vi "armsim-arm-ctrl-init.vi"(11 "Linearsystem":T4) -> (0 "Kalman Error":errorcluster, 1 "KalmanFilter":T3, 2 "LinSysLoopError":bool, 3 "Linear System Loop":T5, 4 "LinearQuadraticRegulator":T1, 6 "Lqr Error":bool)   [LabVIEW 2019]
uses:
  <vilib>/Rock Robotics/WPI/ThirdParty/JAS_Junk/TrajLib/TypeDef/LINEAR_SYSTEM.ctl
  <vilib>/Analysis/Matrix/Datatypes/RealMatrix.ctl
  <vilib>/Rock Robotics/WPI/ThirdParty/JAS_Junk/TrajLib/TypeDef/LINEAR_SYSTEM_LOOP.ctl
  <vilib>/Rock Robotics/WPI/ThirdParty/JAS_Junk/TrajLib/TypeDef/LINEAR_QUADRATIC_REGULATOR.ctl
  <vilib>/Rock Robotics/WPI/ThirdParty/JAS_Junk/TrajLib/TypeDef/LINEAR_PLANT_INV_FF.ctl
  <vilib>/Rock Robotics/WPI/ThirdParty/JAS_Junk/TrajLib/TypeDef/KALMAN_FILTER.ctl
  <vilib>/Rock Robotics/WPI/ThirdParty/JAS_Junk/TrajLib/MatBuilder_Create.vi
  <vilib>/Rock Robotics/WPI/ThirdParty/JAS_Junk/TrajLib/Trajectory_Library.lvlib
  <vilib>/Analysis/Matrix/NI_Matrix.lvlib
panel:
  # "Ref State <States,1>"
  # "Comp and capped \noutput <Inputs,1>"
  # "Controller gain\n<Inputs,States>"
  # "Steady State Gain  \n<States,Outputs>"
  # "State Estimate <Statess,1>"
  # "<States,States>"
  # "<States,Inputs>"
  # "<Outputs,States>"
  # "<Outputs,Inputs>"
  # "<States,1>"
  # "<FUTURE --- CLAMP TYPE -- For now\nuse Normalize>"
  # "Steady State Gain  \n<States,Outputs>"
  # "State Estimate <Statess,1>"
  # "<States,States>"
  # "<States,Inputs>"
  # "<Outputs,States>"
  # "<Outputs,Inputs>"
  # "<States,1>"
  # "<Inputs,1>"
  # "<States,Inputs>"
  # "<States,States>"
  # "Ref State <States,1>"
  # "Comp and capped \noutput <Inputs,1>"
  # "Controller gain\n<Inputs,States>"
  # "<States,States>"
  # "<States,Inputs>"
  # "<Outputs,States>"
  # "<Outputs,Inputs>"
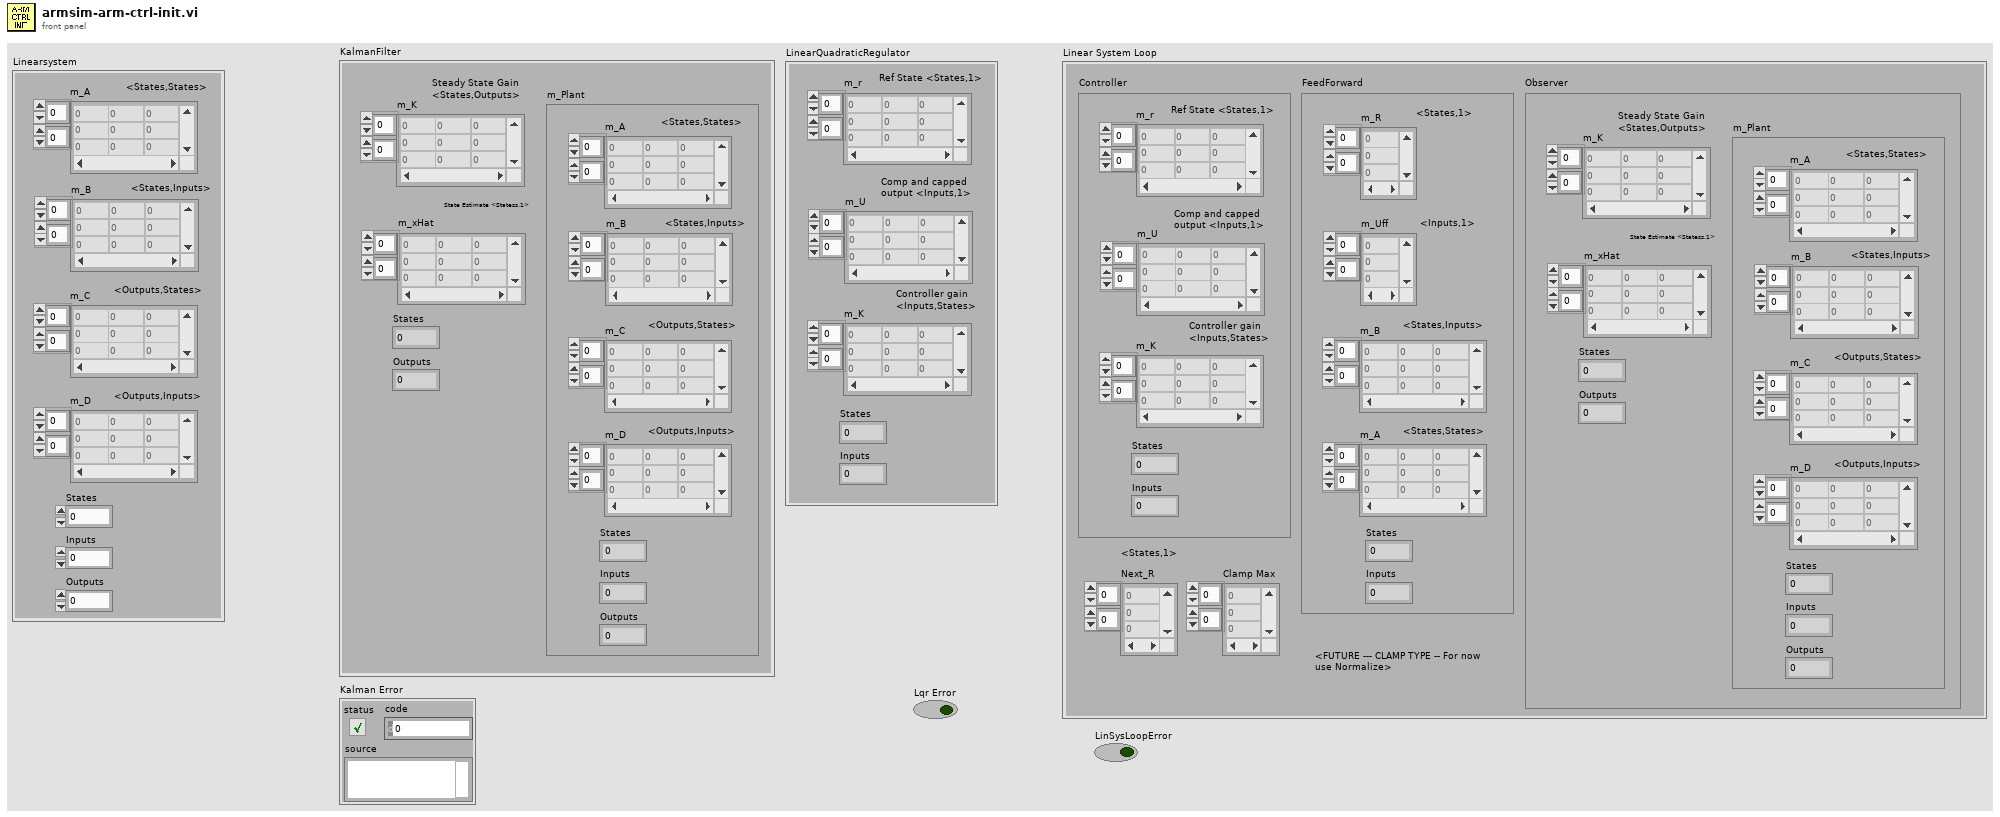
[diagram p1: front panel]
types:
  T1 = typedef "Trajectory_Library.lvlib/LINEAR_QUADRATIC_REGULATOR.ctl" = cluster{"m_r":T2, "m_U":T2, "m_K":T2, "States":i32, "Inputs":i32}
  T2 = typedef "NI_Matrix.lvlib/RealMatrix.ctl" = dbl[][]
  T3 = typedef "Trajectory_Library.lvlib/KALMAN_FILTER.ctl" = cluster{"m_K":T2, "m_xHat":T2, "States":i32, "Outputs":i32, "m_Plant":T4}
  T4 = typedef "Trajectory_Library.lvlib/LINEAR_SYSTEM.ctl" = cluster{"m_A":T2, "m_B":T2, "m_C":T2, "m_D":T2, "States":i32, "Inputs":i32, "Outputs":i32}
  T5 = typedef "Trajectory_Library.lvlib/LINEAR_SYSTEM_LOOP.ctl" = cluster{"Controller":T1, "FeedForward":T6, "Observer":T3, "Next_R":T2, "Clamp Max":T2}
  T6 = typedef "Trajectory_Library.lvlib/LINEAR_PLANT_INV_FF.ctl" = cluster{"m_R":T2, "m_Uff":T2, "m_B":T2, "m_A":T2, "States":i32, "Inputs":i32}
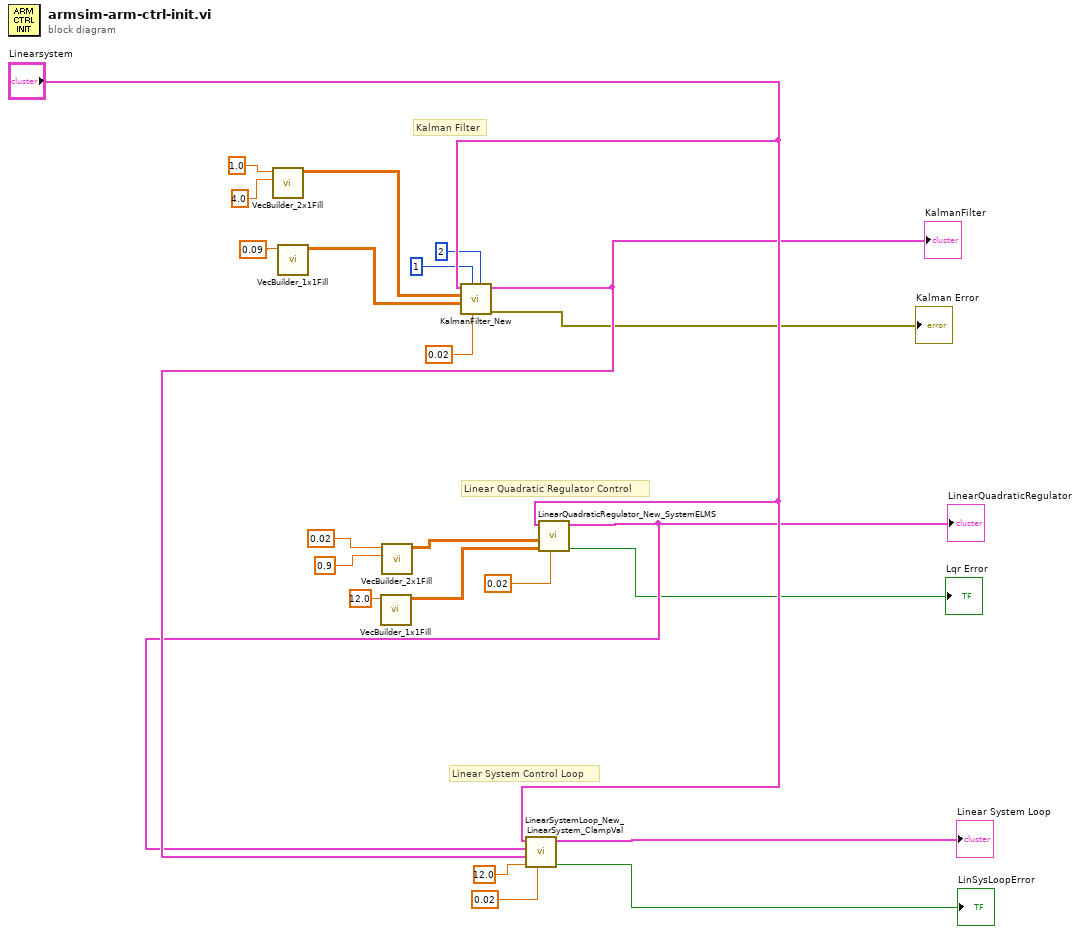
[diagram p0: block diagram]
diagram:
  # "Kalman Filter"
  # "Linear Quadratic Regulator Control"
  # "Linear System Control Loop"
  n1 = call <vilib>:"VecBuilder_2x1Fill.vi"("R1"=4.0, "R0"=1.0 ("R0_C0")) -> ("output matrix"=w11:T2)  [unwired: 9 in]
  n2 = call <vilib>:"VecBuilder_1x1Fill.vi"("R0_C0"=0.09) -> ("output matrix"=w12:T2)  [unwired: 10 in]
  n3 = call <vilib>:"VecBuilder_1x1Fill.vi"("R0_C0"=12.0) -> ("output matrix"=w18:T2)  [unwired: 10 in]
  n4 = call <vilib>:"VecBuilder_2x1Fill.vi"("R1"=0.9 ("R0_C0"), "R0"=0.02 ("R0_C0")) -> ("output matrix"=w16:T2)  [unwired: 9 in]
  n5 = call <vilib>:"KalmanFilter_New.vi"("States"=2, "dt_Seconds"=0.02, "Outputs"=1, "MeasurementStdDevs"=w12, "StateStdDevs"=w11, "Plant"="Linearsystem") -> ("Error"=→"Kalman Error":errorcluster, "KalmanFilter"=w4:T3)  [unwired: 4 in]
  "KalmanFilter" <- w4
  n6 = call <vilib>:"LinearQuadraticRegulator_New_SystemELMS.vi"("dt_Seconds"=0.02, "Relms"=w18, "Qelms"=w16, "LINEARSYSTEM"="Linearsystem") -> ("Error"=→"Lqr Error":bool, "LinearQuadraticRegulator"=w3:T1)  [unwired: 6 in]
  "LinearQuadraticRegulator" <- w3
  n7 = call <vilib>:"LinearSystemLoop_New_LinearSystem_ClampVal.vi"("dT_Seconds"=0.02, "Max_Voltage"=12.0, "Observer"=w4, "Controller"=w3, "Plant"="Linearsystem") -> ("Error"=→"LinSysLoopError":bool, "Linear System Loop"=→"Linear System Loop":T5)  [unwired: 5 in]
